vi "Part 2.vi"(11 "Input":string="714892711431131262132720221453126624699325914653497873272491823531123510909339273820224452407894936892511248875491241226309223658524208482407275183819803893981238951393117621559881306698618296608681543653203748116999546983787150387751297422419423302719228339964412475926361848314117158155489366203640193571778983763559893452555799305618201784647864902896434223677019827554652620895433284524378618964266984994411654262114401369397065429922282240284651137140606858169661297332399986661123648223734045957885756837124716334270256968316689976235699897728581484794946740724336243413561355793014868146474971...") -> (3 "Output":i64)   [LabVIEW 2021]
uses:
  <userlib>/_OpenG.lib/string/string.llb/Convert EOLs (String)__ogtk.vi
panel:
  out "Array":cluster{"Index":i64, "Length":i64}[](array[cluster])
  out "File Map 2":map{i64, cluster{"Index":i64, "Length":i64}}(c390)
  out "File Map":map{i64, cluster{"Index":i64, "Length":i64}}(c390)
  out "Free Space":cluster{"Index":i64, "Length":i64}[](array[cluster])
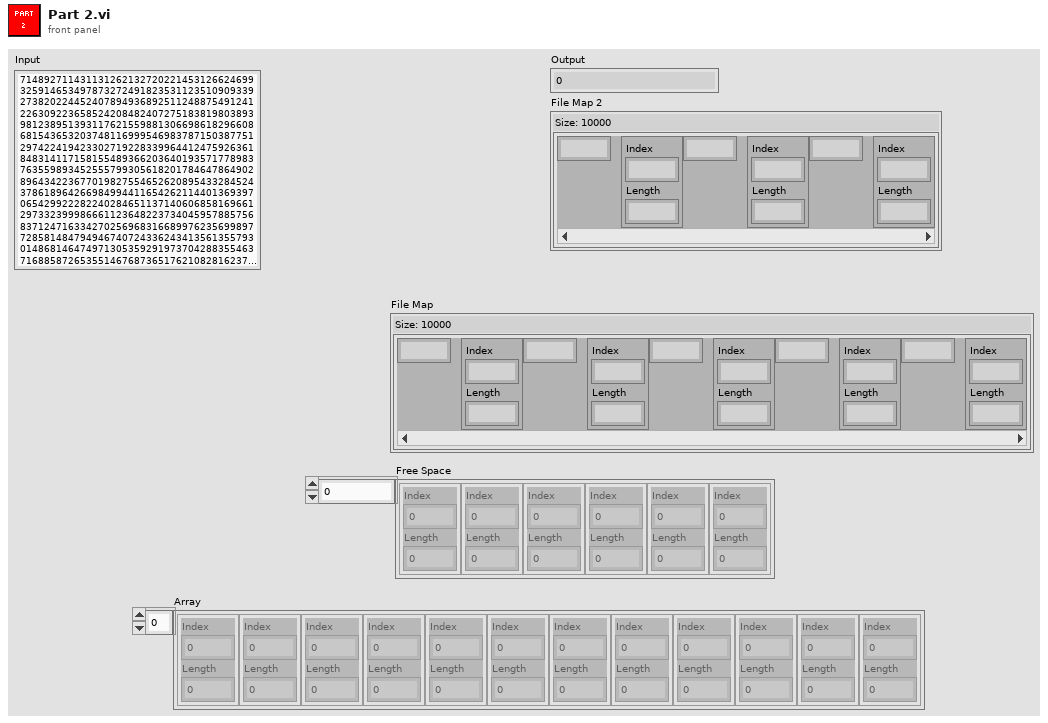
[diagram p1: front panel]
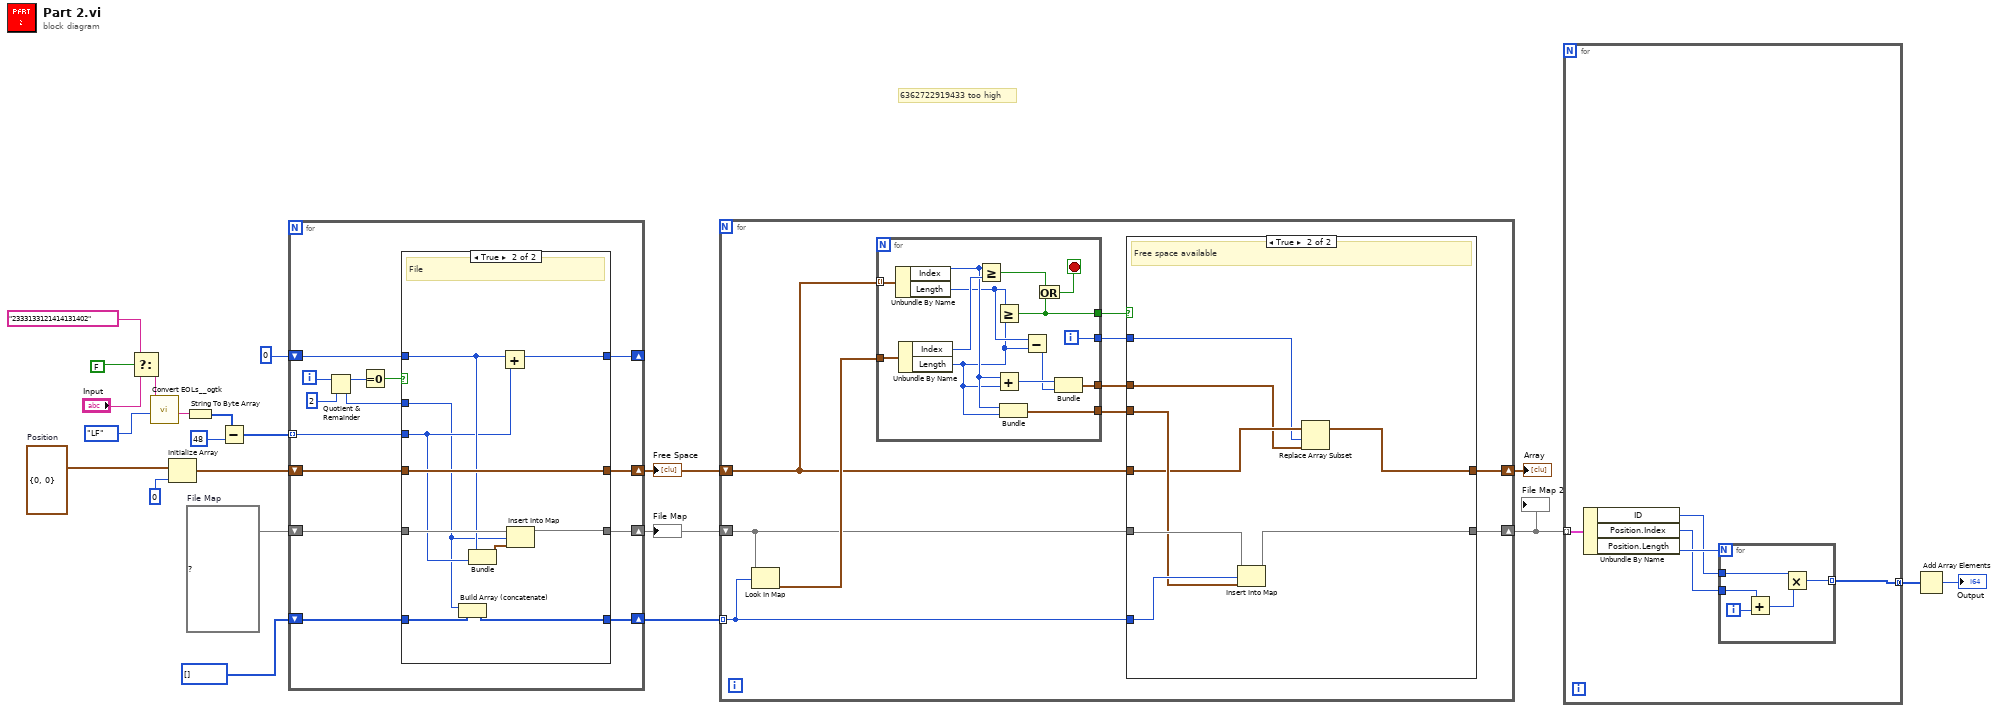
[diagram p0: block diagram]
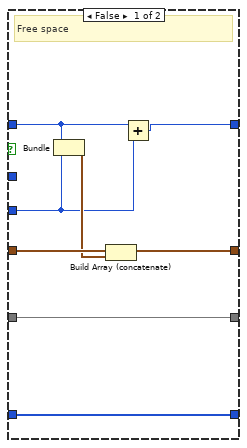
[diagram p3: hidden frame]
diagram:
  w11 = cluster{"Index":i64, "Length":i64} {"Index"=0, "Length"=0}  # Position
  w12 = map{i64, cluster{"Index":i64, "Length":i64}} {}  # File Map
  # "6362722919433 too high"
  n1 = Select(t="2333133121414131402", s=FALSE, f="Input") -> (s? t:f=w15:string)
  n2 = call-poly <userlib>:"Convert EOLs__ogtk.vi"("Convert to:"=enum16{"CR", "LF", "CRLF"}."LF", "String in"=w15) -> ("String out"=w21:string)  [unwired: 9 in]
  n3 = Initialize Array(w11, 0) -> (w9:cluster{"Index":i64, "Length":i64}[])
  n4 = String To Byte Array(string=w21) -> (unsigned byte array=w19:u8[])
  n5 = Subtract(x=w19, y=i64 48) -> (x-y=w18:i64[])
  n6 = for {
    tunnel: w18 -> [w31] mode=indexing
    shift-right: [w25] -> _
    shift-left: i64 0 -> [w30]
    shift-right: [w28] -> w6
    shift-left: w12 -> [w29]
    shift-right: [w26] -> w5
    shift-left: w9 -> [w27]
    shift-right: [w24] -> w7
    shift-left: i64[] [] -> [w23]
    i -> [w36]
    n7 = Quotient & Remainder(x=w36, y=2) -> (x-y*floor(x/y)=w34:i32, floor(x/y)=w32:i32)
    n8 = Equal To 0?(x=w34) -> (x = 0?=w33:bool)
    n9 = case shown="True" w33 {
      tunnel: w32 -> [_ w47]
      tunnel: w31 -> [w39 w49]
      tunnel: w30 -> [w40 w50]
      tunnel: w29 -> [w44 w53]
      tunnel: [w44 w52] -> w28
      tunnel: w27 -> [w43 w54]
      tunnel: [w41 w54] -> w26
      tunnel: [w38 w48] -> w25
      tunnel: [w37 w45] -> w24
      tunnel: w23 -> [w37 w46]
      frame False {
        # "Free space"
        n10 = Bundle(w40, w39) -> (w42:cluster{i64, i64})  [unwired: 1 in]
        n11 = Build Array (concatenate)(w43, w42) -> (w41:cluster{"Index":i64, "Length":i64}[])
        n12 = Add(x=w40, y=w39) -> (x+y=w38:i64)
      }
      frame True {
        # "File"
        n13 = Build Array (concatenate)(w47, w46) -> (w45:i64[])
        n14 = Bundle(w50, w49) -> (w51:cluster{i64, i64})  [unwired: 1 in]
        n15 = Add(x=w50, y=w49) -> (x+y=w48:i64)
        n16 = Insert Into Map(map in=w53, key=w47, value=w51) -> (map out=w52:map{i64, cluster{"Index":i64, "Length":i64}})  [unwired: 2 out]
      }
    }
  }
  "Free Space" <- w5
  "File Map" <- w6
  n17 = for {
    tunnel: w7 -> [w58] mode=indexing
    shift-right: [w60] -> w1
    shift-left: w5 -> [w62]
    shift-right: [w59] -> w4
    shift-left: w6 -> [w61]
    n18 = Look In Map(map=w61, key=w58) -> (value=w64:cluster{"Index":i64, "Length":i64})  [unwired: 1 in, 1 out]
    n19 = for {
      tunnel: w62 -> [w88] mode=indexing
      tunnel: w64 -> [w87]
      tunnel: [w83] -> w63
      tunnel: [w82] -> w57
      tunnel: [w77] -> w56
      tunnel: [w76] -> w55
      i -> [w76]
      stop <- w84 stop-if-true
      n20 = Unbundle By Name(w88) -> ("Index"=w81:i64, "Length"=w79:i64)
      n21 = Unbundle By Name(w87) -> ("Index"=w86:i64, "Length"=w78:i64)
      n22 = Greater Or Equal?(x=w81, y=w86) -> (x >= y?=w85:bool)
      n23 = Greater Or Equal?(x=w79, y=w78) -> (x >= y?=w83:bool)
      n24 = Add(x=w81, y=w78) -> (x+y=w80:i64)
      n25 = Bundle("Index"=w81, "Length"=w78) -> (w82:cluster{"Index":i64, "Length":i64})  [unwired: 1 in]
      n26 = Subtract(x=w79, y=w78) -> (x-y=w75:i64)
      n27 = Or(x=w85, y=w83) -> (x .or. y?=w84:bool)
      n28 = Bundle(w80, w75) -> (w77:cluster{i64, i64})  [unwired: 1 in]
    }
    n29 = case shown="True" w63 {
      tunnel: w62 -> [w66 w70]
      tunnel: w61 -> [w65 w74]
      tunnel: [w66 w68] -> w60
      tunnel: [w65 w71] -> w59
      tunnel: w58 -> [_ w73]
      tunnel: w57 -> [_ w72]
      tunnel: w56 -> [_ w67]
      tunnel: w55 -> [_ w69]
      frame False {
        # "No free space available"
      }
      frame True {
        # "Free space available"
        n30 = Insert Into Map(map in=w74, key=w73, value=w72) -> (map out=w71:map{i64, cluster{"Index":i64, "Length":i64}})  [unwired: 2 out]
        n31 = Replace Array Subset(array=w70, new element=w67, index=w69) -> (w68:cluster{"Index":i64, "Length":i64}[])
      }
    }
  }
  "File Map 2" <- w4
  "Array" <- w1
  n32 = for {
    tunnel: w4 -> [w93] mode=indexing
    tunnel: [w89] -> w3 mode=concatenating
    n33 = Unbundle By Name(w93) -> ("ID"=w91:i64, "Position.Index"=w90:i64, "Position.Length"=w92:i64)
    n34 = for {
      N: w92 -> [_]
      tunnel: w91 -> [w95]
      tunnel: w90 -> [w97]
      tunnel: [w94] -> w89 mode=indexing
      i -> [w98]
      n35 = Add(x=w97, y=w98) -> (x+y=w96:i64)
      n36 = Multiply(x=w95, y=w96) -> (x*y=w94:i64)
    }
  }
  n37 = Add Array Elements(numeric array=w3) -> (sum=→"Output":i64)
